vi "MLPut.vi"(1 "End":bool, 2 "Variant":variant, 3 "mlp in":u64) -> (0 "mlp out":u64)   [LabVIEW 2014]
uses:
  <vilib>/Utility/VariantDataType/Type.ctl
  <vilib>/Utility/VariantDataType/VariantType.lvlib
  ml64i4.dll
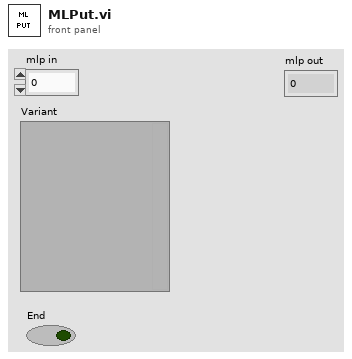
[diagram p1: front panel]
types:
  T1 = typedef "VariantType.lvlib/Type.ctl" = enum8{"Invalid Type", "Void", "I8", "I16", "I32", "I64", "U8", "U16", "U32", "U64", "Single Float", "Double Float", "Extended Float", "Single Complex", "Double Complex", "Extended Complex", "Enum U8", "Enum U16", "Enum U32", "Enum U64", "Single Float With Unit", "Double Float With Unit", "Extended Float With Unit", "Single Complex with Unit", "Double Complex with Unit", "Extended Complex with Unit", "Boolean", "String", "Path", "Picture", "Tag", "Array", "Cluster", "Variant", "LV Variant", "Waveform", "Timestamp", "Digital Waveform", "Digital Data", "ExpressData", "Refnum", "External Data", "VI", "Poly VI", "LabVIEW Class Instance", "Fixed Point"}
  T2 = typedef "VariantType.lvlib/RefnumType.ctl" = enum16{"NotARefnum", "UnknownRefnum", "Generic", "Datalog", "ByteStream", "Device", "Occurence", "TCPNetConnection", "Auto", "Menu", "Imaq", "Hardware", "DataSocket", "Visa", "IVI", "UDPNetConnection", "Notifier", "Queue", "Irda", "EventReg", "DotNet", "UserEvent", "Callback", "UNUSED_EMPTY_POSITION", "BlueToothNetConnection", "LVObjApp", "LVObjVI", "LVObjUnknown", "GenericClass", "UserDefinedRefnumTag", "DataValue", "RT FIFO", "TDMS File"}
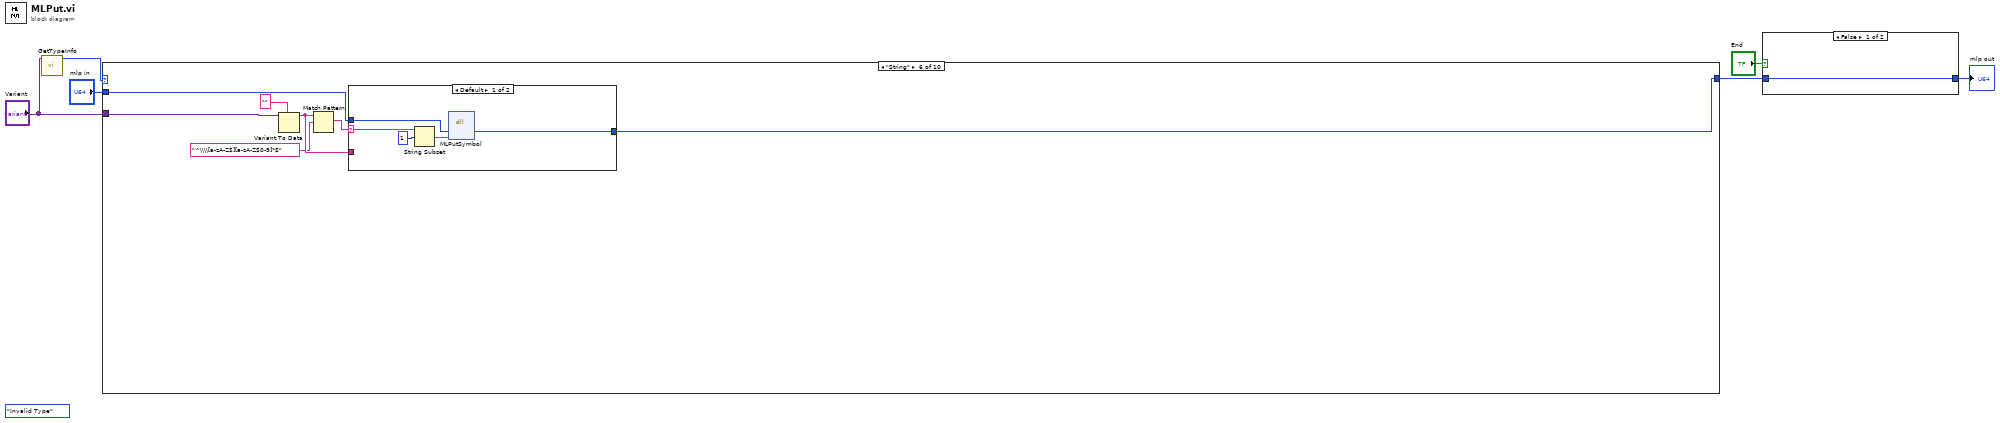
[diagram p0: block diagram]
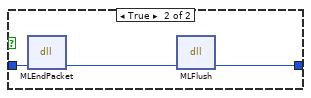
[diagram p2: hidden frame]
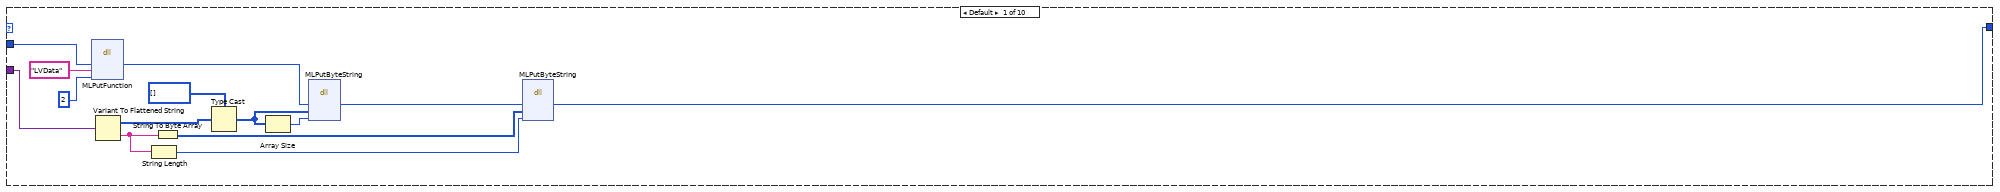
[diagram p3: hidden frame]
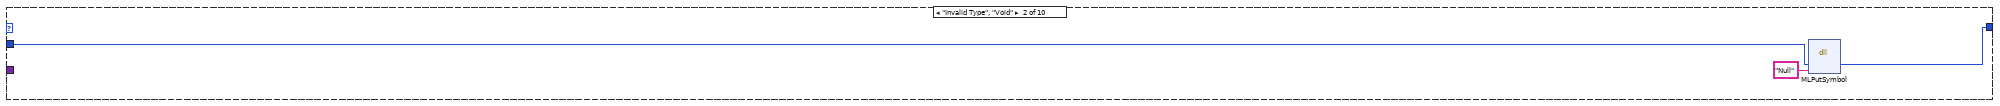
[diagram p4: hidden frame]
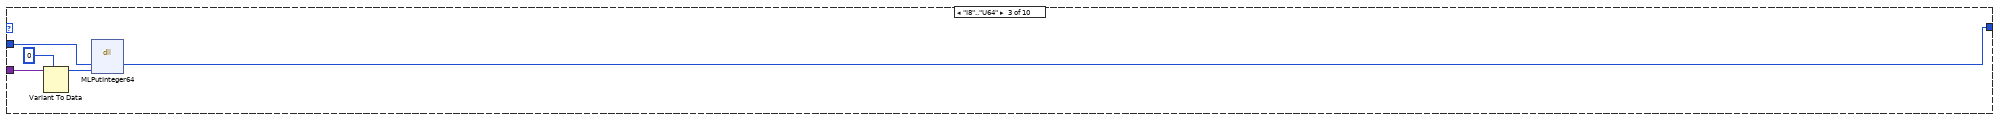
[diagram p5: hidden frame]
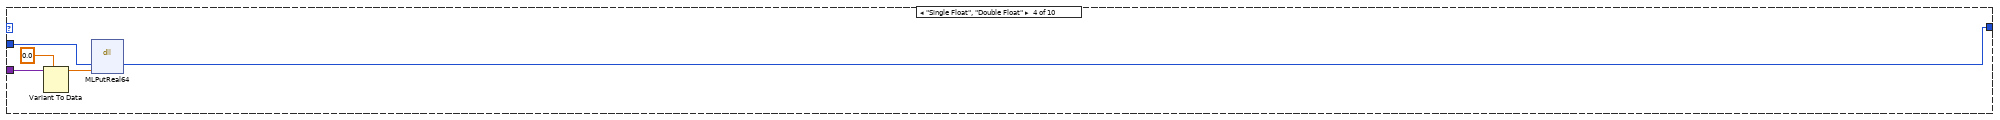
[diagram p6: hidden frame]
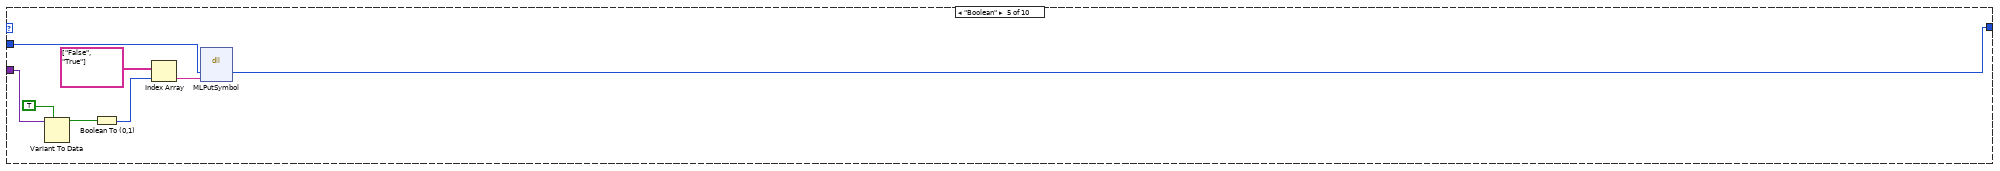
[diagram p7: hidden frame]
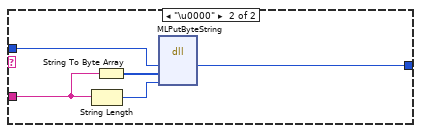
[diagram p8: hidden frame]
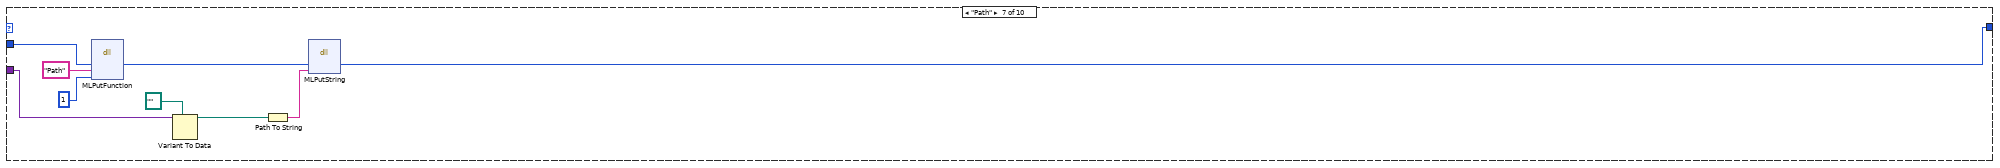
[diagram p9: hidden frame]
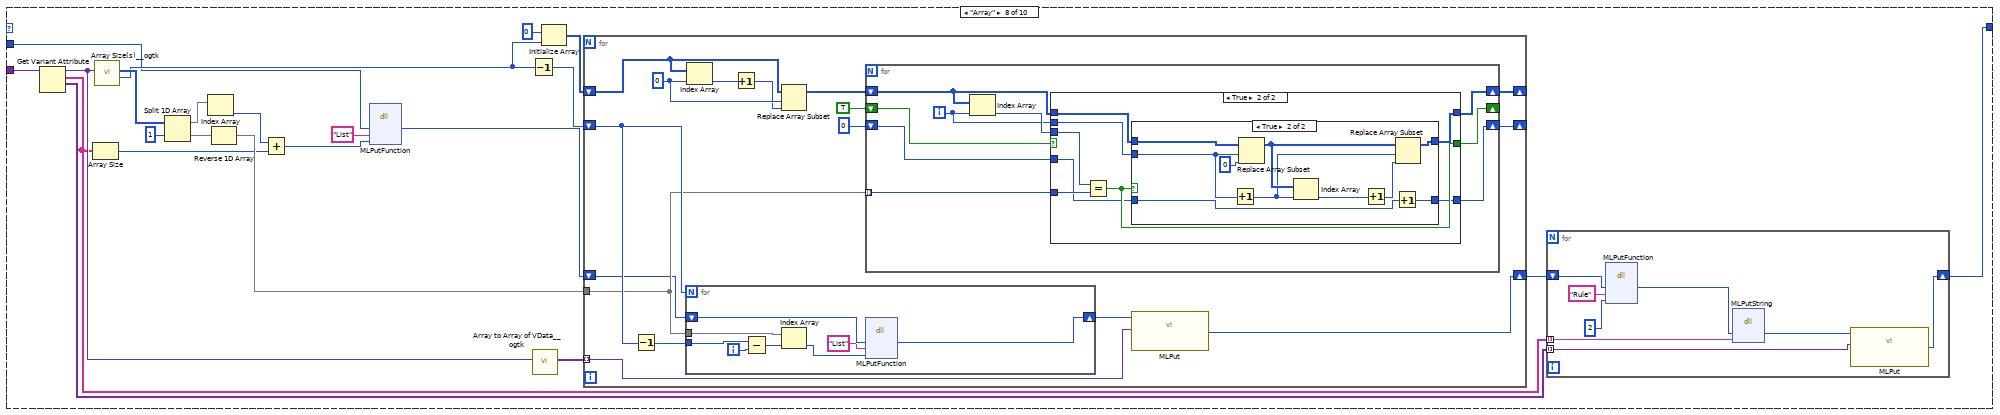
[diagram p10: hidden frame]
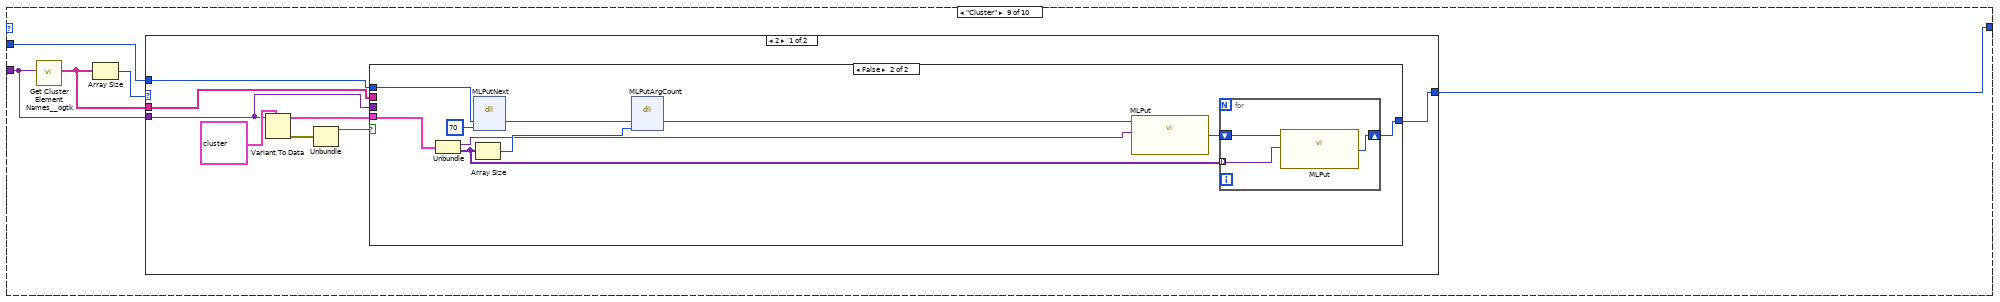
[diagram p13: hidden frame]
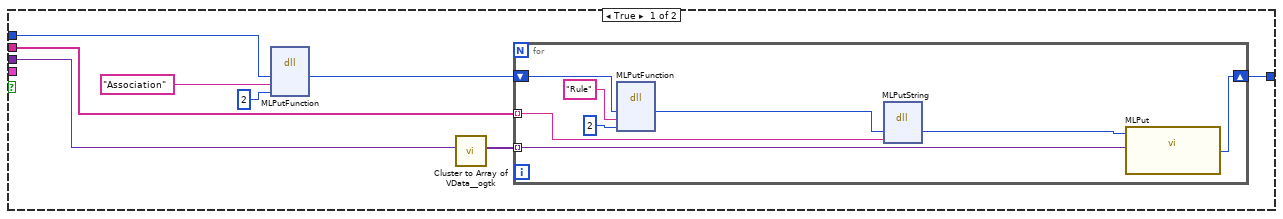
[diagram p14: hidden frame]
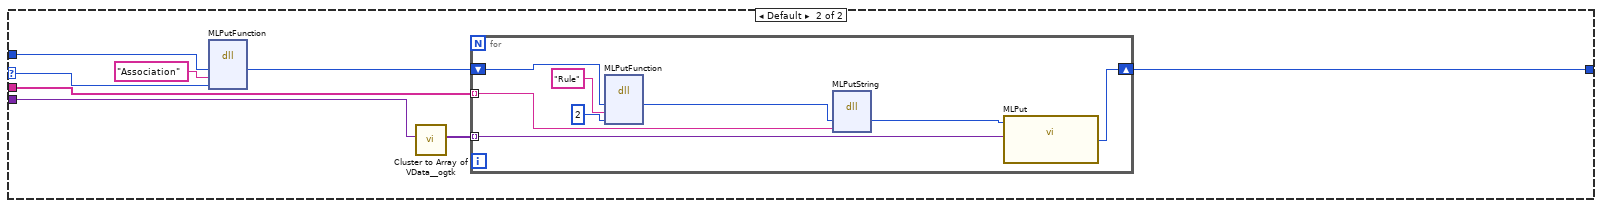
[diagram p15: hidden frame]
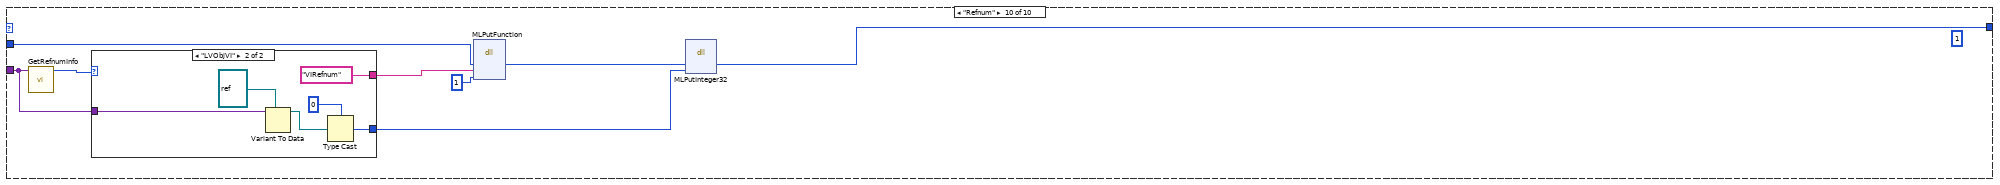
[diagram p16: hidden frame]
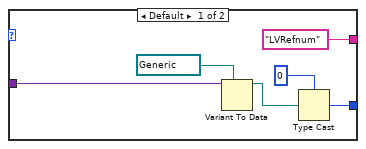
[diagram p17: hidden frame]
diagram:
  (unwired) Type."Invalid Type" ("Type Enum")
  n1 = call <vilib>:"GetTypeInfo.vi"("Variant"="Variant") -> ("Type Enum"=w6:T1)  [unwired: 6 in, 4 out]
  n2 = case shown="\"String\"" w6 {
    tunnel: "mlp in" -> [w15 w22 w25 w31 w37 w46 w62 w79 w156 w217]
    tunnel: "Variant" -> [w20 _ w28 w33 w41 w48 w67 w76 w154 w218]
    tunnel: [w7 w23 w24 w30 w38 w45 w61 w68 w158 w214] -> w3
    frame Default {
      n3 = dll-call lib="ml64i4.dll" fn="MLPutFunction"("mlp"=w15, "s"="LVData", "argc"=2) -> ("mlp"=w10:u64)  [unwired: 6 in, 2 out]
      n4 = Variant To Flattened String(Variant=w20) -> (data string=w12:string, 1:w19:i16[])
      n5 = String Length(string=w12) -> (length=w14:i32)
      n6 = String To Byte Array(string=w12) -> (unsigned byte array=w13:u8[])
      n7 = Type Cast(type=u8[] [], x=w19) -> (*(type *) &x=w8:u8[])
      n8 = Array Size(array=w8) -> (size(s)=w9:i32)
      n9 = dll-call lib="ml64i4.dll" fn="MLPutByteString"("mlp"=w10, "s"=w8, "len"=w9) -> ("mlp"=w11:u64)  [unwired: 6 in, 2 out]
      n10 = dll-call lib="ml64i4.dll" fn="MLPutByteString"("mlp"=w11, "s"=w13, "len"=w14) -> ("mlp"=w7:u64)  [unwired: 6 in, 2 out]
    }
    frame "Invalid Type", "Void" {
      n11 = dll-call lib="ml64i4.dll" fn="MLPutSymbol"("mlp"=w22, "s"="Null") -> ("mlp"=w23:u64)  [unwired: 5 in, 2 out]
    }
    frame "I8".."U64" {
      n12 = Variant To Data(type=i64 0 ("n"), Variant=w28) -> (data=w26:i64)  [unwired: 1 in, 1 out]
      n13 = dll-call lib="ml64i4.dll" fn="MLPutInteger64"("mlp"=w25, "w"=w26) -> ("mlp"=w24:u64)  [unwired: 5 in, 2 out]
    }
    frame "Single Float", "Double Float" {
      n14 = Variant To Data(type=0.0 ("n"), Variant=w33) -> (data=w29:dbl)  [unwired: 1 in, 1 out]
      n15 = dll-call lib="ml64i4.dll" fn="MLPutReal64"("mlp"=w31, "d"=w29) -> ("mlp"=w30:u64)  [unwired: 5 in, 2 out]
    }
    frame "Boolean" {
      n16 = Variant To Data(type=TRUE, Variant=w41) -> (data=w39:bool)  [unwired: 1 in, 1 out]
      n17 = Boolean To (0,1)(Boolean=w39) -> (0, 1=w35:i16)
      n18 = Index Array(array=string[] ["False", "True"], index=w35) -> (element=w34:string)
      n19 = dll-call lib="ml64i4.dll" fn="MLPutSymbol"("mlp"=w37, "s"=w34) -> ("mlp"=w38:u64)  [unwired: 5 in, 2 out]
    }
    frame "String" {
      n20 = Variant To Data(type="", Variant=w48) -> (data=w44:string)  [unwired: 1 in, 1 out]
      n21 = Match Pattern(string=w44, regular expression="^\\\\[a-zA-Z$][a-zA-Z$0-9]*$") -> (match substring=w42:string)  [unwired: 1 in, 3 out]
      n22 = case shown="Default" w42 {
        selector: w42 -> [w51 _]
        tunnel: w46 -> [w53 w58]
        tunnel: [w52 w55] -> w45
        tunnel: w44 -> [_ w54]
        frame Default {
          n23 = String Subset(string=w51, offset (0)=1) -> (substring=w49:string)  [unwired: 1 in]
          n24 = dll-call lib="ml64i4.dll" fn="MLPutSymbol"("mlp"=w53, "s"=w49) -> ("mlp"=w52:u64)  [unwired: 5 in, 2 out]
        }
        frame "\u0000" {
          n25 = String Length(string=w54) -> (length=w57:i32)
          n26 = String To Byte Array(string=w54) -> (unsigned byte array=w56:u8[])
          n27 = dll-call lib="ml64i4.dll" fn="MLPutByteString"("mlp"=w58, "s"=w56, "len"=w57) -> ("mlp"=w55:u64)  [unwired: 6 in, 2 out]
        }
      }
    }
    frame "Path" {
      n28 = dll-call lib="ml64i4.dll" fn="MLPutFunction"("mlp"=w62, "s"="Path", "argc"=1) -> ("mlp"=w63:u64)  [unwired: 6 in, 2 out]
      n29 = Variant To Data(type=path "" ("path"), Variant=w67) -> (data=w65:path)  [unwired: 1 in, 1 out]
      n30 = Path To String(path=w65) -> (string=w64:string)
      n31 = dll-call lib="ml64i4.dll" fn="MLPutString"("mlp"=w63, "s"=w64) -> ("mlp"=w61:u64)  [unwired: 5 in, 2 out]
    }
    frame "Array" {
      n32 = Get Variant Attribute(Variant=w76) -> (duplicate Variant=w75:variant, names=w70:string[], values=w71:variant[])  [unwired: 3 in, 1 out]
      n33 = Array Size(array=w70) -> (size(s)=w74:i32)
      n34 = call <userlib>:"Array Size(s)__ogtk.vi"("Array"=w75) -> ("N dims"=w82:u32, "Size(s)"=w83:u32[])  [unwired: 8 in, 1 out]
      n35 = Split 1D Array(array=w83, index=1) -> (first subarray=w80:u32[], second subarray=w85:u32[])
      n36 = Index Array(array=w80) -> (element=w73:u32)  [unwired: 1 in]
      n37 = Reverse 1D Array(array=w85) -> (reversed array=w86:u32[])
      n38 = Add(x=w73, y=w74) -> (x+y=w72:u32)
      n39 = dll-call lib="ml64i4.dll" fn="MLPutFunction"("mlp"=w79, "s"="List", "argc"=w72) -> ("mlp"=w77:u64)  [unwired: 6 in, 2 out]
      n40 = Decrement(x=w82) -> (x-1=w81:u32)
      n41 = call <userlib>:"Array to Array of VData__ogtk.vi"("MultiD Array"=w75) -> ("1D Array of Variants"=w89:variant[])  [unwired: 9 in, 1 out]
      n42 = Initialize Array(0 ("nrec"), w82) -> (w87:i32[])
      n43 = for {
        tunnel: w89 -> [w98] mode=indexing
        shift-right: [w104] -> _
        shift-left: w87 -> [w113]
        tunnel: w86 -> [w105]
        shift-right: [w103] -> _
        shift-left: w81 -> [w111]
        shift-right: [w99] -> w69
        shift-left: w77 -> [w100]
        w109 = 0 ("index")
        n44 = Decrement(x=w111) -> (x-1=w112:u32)
        n45 = for {
          N: w111 -> [_]
          shift-right: [w148] -> w107
          shift-left: w100 -> [w149]
          tunnel: w105 -> [w153]
          tunnel: w112 -> [w150]
          i -> [w152]
          n46 = Subtract(x=w150, y=w152) -> (x-y=w151:u32)
          n47 = Index Array(array=w153, index=w151) -> (element=w147:u32)
          n48 = dll-call lib="ml64i4.dll" fn="MLPutFunction"("mlp"=w149, "s"="List", "argc"=w147) -> ("mlp"=w148:u64)  [unwired: 6 in, 2 out]
        }
        n49 = Index Array(array=w113, index=w109) -> (element=w110:i32)
        n50 = Increment(x=w110) -> (x+1=w108:i32)
        n51 = Replace Array Subset(array=w113, new element=w108, index=w109) -> (w106:i32[])
        n52 = for {
          shift-right: [w116] -> w104
          shift-left: w106 -> [w118]
          tunnel: w105 -> [w120] mode=indexing
          shift-right: [w119] -> _
          shift-left: TRUE -> [w122]
          shift-right: [w114] -> w103
          shift-left: 0 ("new element/subarray") -> [w115]
          i -> [w117]
          n53 = Index Array(array=w118, index=w117) -> (element=w121:i32)
          n54 = case shown="True" w122 {
            selector: w122 -> [w125 _]
            tunnel: [w124 w133] -> w116
            tunnel: w121 -> [_ w132]
            tunnel: w120 -> [_ w131]
            tunnel: [w125 w130] -> w119
            tunnel: w118 -> [w124 w129]
            tunnel: w117 -> [_ w128]
            tunnel: w115 -> [w123 w127]
            tunnel: [w123 w126] -> w114
            frame False {
            }
            frame True {
              n55 = Equal?(x=w132, y=w131) -> (x = y?=w130:bool)
              n56 = case shown="True" w130 {
                tunnel: [w135 w140] -> w133
                tunnel: w129 -> [w135 w143]
                tunnel: w128 -> [_ w142]
                tunnel: w127 -> [w134 w137]
                tunnel: [w134 w136] -> w126
                frame False {
                }
                frame True {
                  n57 = Increment(x=w142) -> (x+1=w139:i32)
                  n58 = Replace Array Subset(array=w143, new element=0 ("new element/subarray"), index=w142) -> (w141:i32[])
                  n59 = Index Array(array=w141, index=w139) -> (element=w144:i32)
                  n60 = Increment(x=w144) -> (x+1=w138:i32)
                  n61 = Increment(x=w137) -> (x+1=w136:i32)
                  n62 = Replace Array Subset(array=w141, new element=w138, index=w139) -> (w140:i32[])
                }
              }
            }
          }
        }
        n63 = call "MLPut.vi"("Variant"=w98, "mlp in"=w107) -> ("mlp out"=w99:u64)  [unwired: 1 in]
      }
      n64 = for {
        tunnel: w71 -> [w91] mode=indexing
        tunnel: w70 -> [w90] mode=indexing
        shift-right: [w97] -> w68
        shift-left: w69 -> [w94]
        n65 = dll-call lib="ml64i4.dll" fn="MLPutFunction"("mlp"=w94, "s"="Rule", "argc"=2) -> ("mlp"=w93:u64)  [unwired: 6 in, 2 out]
        n66 = dll-call lib="ml64i4.dll" fn="MLPutString"("mlp"=w93, "s"=w90) -> ("mlp"=w92:u64)  [unwired: 5 in, 2 out]
        n67 = call "MLPut.vi"("Variant"=w91, "mlp in"=w92) -> ("mlp out"=w97:u64)  [unwired: 1 in]
      }
    }
    frame "Cluster" {
      n68 = call <userlib>:"Get Cluster Element Names__ogtk.vi"("Cluster"=w154) -> ("Element Names"=w155:string[])  [unwired: 9 in, 1 out]
      n69 = Array Size(array=w155) -> (size(s)=w157:i32)
      n70 = case shown="2" w157 {
        selector: w157 -> [_ w200]
        tunnel: [w165 w203] -> w158
        tunnel: w156 -> [w166 w199]
        tunnel: w155 -> [w160 w202]
        tunnel: w154 -> [w159 w197]
        frame 2 {
          n71 = Variant To Data(type=cluster{"Variant":variant, variant[]} {"Variant"=variant, []} ("output cluster"), Variant=w159) -> (data=w163:cluster{"Variant":variant, variant[]}, error out=w162:errorcluster)  [unwired: 1 in]
          n72 = Unbundle(w162) -> ("status"=w161:bool)  [unwired: 2 out]
          n73 = case shown="False" w161 {
            tunnel: w166 -> [w173 w190]
            tunnel: [w168 w186] -> w165
            tunnel: w163 -> [_ w185]
            tunnel: w160 -> [w169 _]
            tunnel: w159 -> [w167 _]
            frame True {
              n74 = dll-call lib="ml64i4.dll" fn="MLPutFunction"("mlp"=w173, "s"="Association", "argc"=2) -> ("mlp"=w170:u64)  [unwired: 6 in, 2 out]
              n75 = call <userlib>:"Cluster to Array of VData__ogtk.vi"("Cluster"=w167) -> ("Array of VData"=w171:variant[])  [unwired: 9 in, 1 out]
              n76 = for {
                tunnel: w169 -> [w175] mode=indexing
                shift-right: [w182] -> w168
                shift-left: w170 -> [w178]
                tunnel: w171 -> [w176] mode=indexing
                n77 = dll-call lib="ml64i4.dll" fn="MLPutFunction"("mlp"=w178, "s"="Rule", "argc"=2) -> ("mlp"=w179:u64)  [unwired: 6 in, 2 out]
                n78 = dll-call lib="ml64i4.dll" fn="MLPutString"("mlp"=w179, "s"=w175) -> ("mlp"=w177:u64)  [unwired: 5 in, 2 out]
                n79 = call "MLPut.vi"("Variant"=w176, "mlp in"=w177) -> ("mlp out"=w182:u64)  [unwired: 1 in]
              }
            }
            frame False {
              n80 = Unbundle(w185) -> ("Variant"=w183:variant, w184:variant[])
              n81 = dll-call lib="ml64i4.dll" fn="MLPutNext"("mlp"=w190, "tok"=70) -> ("mlp"=w191:u64)  [unwired: 5 in, 2 out]
              n82 = Array Size(array=w184) -> (size(s)=w192:i32)
              n83 = dll-call lib="ml64i4.dll" fn="MLPutArgCount"("mlp"=w191, "argc"=w192) -> ("mlp"=w188:u64)  [unwired: 5 in, 2 out]
              n84 = call "MLPut.vi"("Variant"=w183, "mlp in"=w188) -> ("mlp out"=w187:u64)  [unwired: 1 in]
              n85 = for {
                shift-right: [w193] -> w186
                shift-left: w187 -> [w194]
                tunnel: w184 -> [w195] mode=indexing
                n86 = call "MLPut.vi"("Variant"=w195, "mlp in"=w194) -> ("mlp out"=w193:u64)  [unwired: 1 in]
              }
            }
          }
        }
        frame Default {
          n87 = dll-call lib="ml64i4.dll" fn="MLPutFunction"("mlp"=w199, "s"="Association", "argc"=w200) -> ("mlp"=w198:u64)  [unwired: 6 in, 2 out]
          n88 = call <userlib>:"Cluster to Array of VData__ogtk.vi"("Cluster"=w197) -> ("Array of VData"=w196:variant[])  [unwired: 9 in, 1 out]
          n89 = for {
            tunnel: w202 -> [w204] mode=indexing
            shift-right: [w211] -> w203
            shift-left: w198 -> [w207]
            tunnel: w196 -> [w205] mode=indexing
            n90 = dll-call lib="ml64i4.dll" fn="MLPutFunction"("mlp"=w207, "s"="Rule", "argc"=2) -> ("mlp"=w208:u64)  [unwired: 6 in, 2 out]
            n91 = dll-call lib="ml64i4.dll" fn="MLPutString"("mlp"=w208, "s"=w204) -> ("mlp"=w206:u64)  [unwired: 5 in, 2 out]
            n92 = call "MLPut.vi"("Variant"=w205, "mlp in"=w206) -> ("mlp out"=w211:u64)  [unwired: 1 in]
          }
        }
      }
    }
    frame "Refnum" {
      (unwired) 1 ("narr")
      n93 = call <vilib>:"GetRefnumInfo.vi"("Variant"=w218) -> ("ReferenceType"=w219:T2)  [unwired: 7 in, 3 out]
      n94 = case shown="\"LVObjVI\"" w219 {
        tunnel: w218 -> [w225 w230]
        tunnel: [w221 w227] -> w215
        tunnel: ["LVRefnum" ("str") "VIRefnum" ("str")] -> w213
        frame Default {
          n95 = Variant To Data(type=refnum<vi> refnum ("reference"), Variant=w225) -> (data=w223:refnum<vi>)  [unwired: 1 in, 1 out]
          n96 = Type Cast(type=u32 0 ("i"), x=w223) -> (*(type *) &x=w221:u32)
        }
        frame "LVObjVI" {
          n97 = Variant To Data(type=refnum<vi> refnum ("vi reference"), Variant=w230) -> (data=w229:refnum<vi>)  [unwired: 1 in, 1 out]
          n98 = Type Cast(type=u32 0 ("i"), x=w229) -> (*(type *) &x=w227:u32)
        }
      }
      n99 = dll-call lib="ml64i4.dll" fn="MLPutFunction"("mlp"=w217, "s"=w213, "argc"=1) -> ("mlp"=w216:u64)  [unwired: 6 in, 2 out]
      n100 = dll-call lib="ml64i4.dll" fn="MLPutInteger32"("mlp"=w216, "i"=w215) -> ("mlp"=w214:u64)  [unwired: 5 in, 2 out]
    }
  }
  n101 = case shown="False" "End" {
    tunnel: w3 -> [w232 w234]
    tunnel: [w232 w233] -> w2
    frame False {
    }
    frame True {
      n102 = dll-call lib="ml64i4.dll" fn="MLEndPacket"("mlp"=w234) -> ("mlp"=w235:u64)  [unwired: 4 in, 2 out]
      n103 = dll-call lib="ml64i4.dll" fn="MLFlush"("mlp"=w235) -> ("mlp"=w233:u64)  [unwired: 4 in, 2 out]
    }
  }
  "mlp out" <- w2
